vi "Signal Processing.vi"(0 "Vessel in":refnum<class "Vessel.lvclass">, 5 "error in (no error)":errorcluster) -> (14 "Vessel out":refnum<class "Vessel.lvclass">, 19 "error out":errorcluster)   [LabVIEW 2014, in "Vessel.lvclass"]
uses:
  Vessel.lvclass
  Vessel.lvclass/Vessel.ctl
  Supervisor/Supervisor.lvclass
  Sensor/Sensor.lvclass
panel:
  in  "T_dvl":dbl[](array[numeric])=[0.0, 0.0, 45.0]
  in  "Manual Sensor\nPosition Override":bool
  in  "r_dvl":dbl[](array[numeric])=[0.46, -0.5, 0.0]
  in  "r_tp":dbl[](array[numeric])=[1.35, 0.15, 0.0]
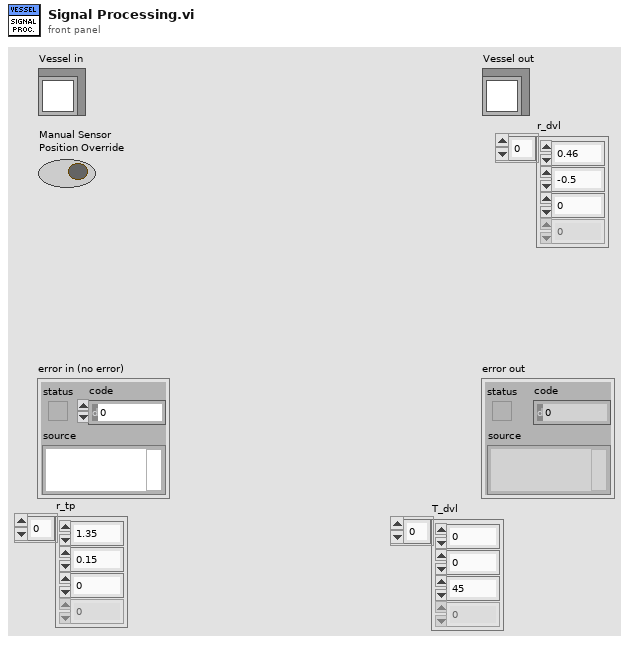
[diagram p1: front panel]
types:
  T1 = cluster{"Measured":cluster{"Eta":dbl[], "Nu":dbl[], "Eta Dot":dbl[], "Nu Dot":dbl[]}, "Estimated":cluster{"Eta":dbl[], "Nu":dbl[], "Eta Dot":dbl[], "Nu Dot":dbl[]}, "Desired":cluster{"Eta":dbl[], "Nu":dbl[], "Eta Dot":dbl[], "Nu Dot":dbl[]}, "Previous Desired":cluster{"Eta":dbl[], "Nu":dbl[], "Eta Dot":dbl[], "Nu Dot":dbl[]}, "tau":dbl[], "Altitude":cluster{"Measured":dbl, "Estimated":dbl, "Desired":dbl, "Previous Desired":dbl, "Approximated":dbl, "grad F":dbl[]}, "rpm":dbl[], "Attitude":cluster{"Theta Measured":dbl[], "Theta Estimated":dbl[], "Omega Measured":dbl[], "Omega Estimated":dbl[], "Gyro Bias":dbl[]}}
  T2 = cluster{"Set Origin":bool, "New WP":bool, "Types of Change":enum16{"Current NED", "Change NED"}, "Make Change":bool, "Optimal Heading":bool, "New SetPoint":cluster{"North":dbl, "East":dbl, "Depth":dbl, "Heading":dbl}, "Update Reference":cluster{"Mode Change":bool, "Current Position":dbl[]}, "Go":bool, "Go heading":bool}
  T3 = cluster{"Sensor Drop Out":dbl[], "Sensor Health":bool[]}
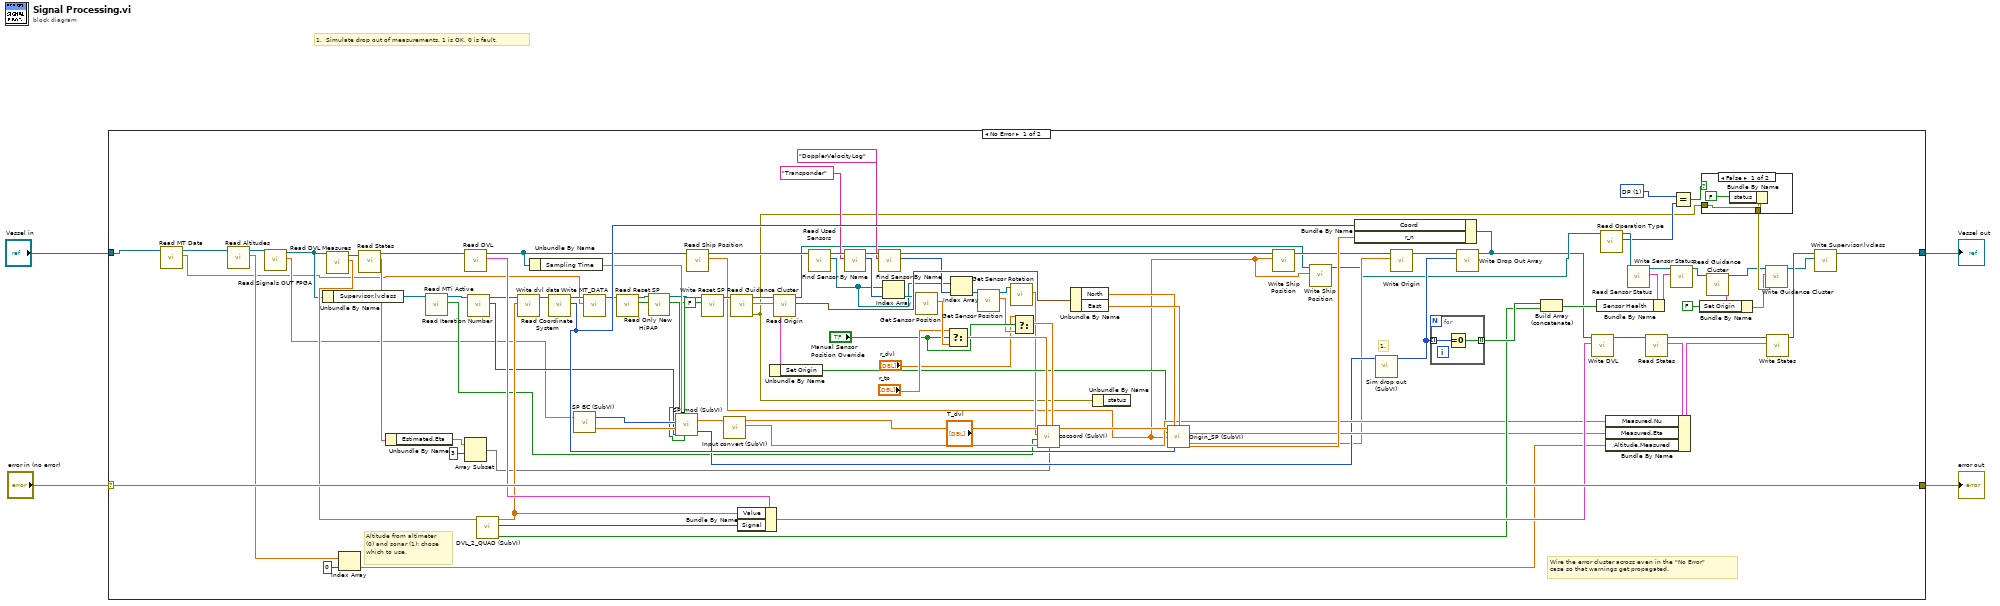
[diagram p0: block diagram]
diagram:
  # "1.  Simulate drop out of measurements. 1 is OK, 0 is fault."
  n1 = case shown="No Error" "error in (no error)" {
    selector: "error in (no error)" -> [w110 w118]
    tunnel: [w110 w118] -> w3
    tunnel: [w103 w117] -> w1
    tunnel: "Vessel in" -> [w18 w117]
    frame No Error {
      w84 = u16 1 items=["Tracking", "DP", "Joystick"] ("Operation Type")
      # "1."
      # "Altitude from altimeter (0) and sonar (1): chose which to use."
      # "Wire the error cluster across even in the \"No Error\"\ncase so that warnings get propagated."
      n2 = call-dynamic "Read MT Data.vi"("Vessel in"=w18) -> ("MT Data"=w16:sgl[], "Vessel out"=w17:refnum<class "Vessel.lvclass">)  [unwired: 8 in, 1 out]
      n3 = call-dynamic "Read Altitudes.vi"("Vessel in"=w17) -> ("Altitudes"=w19:dbl[], "Vessel out"=w20:refnum<class "Vessel.lvclass">)  [unwired: 8 in, 1 out]
      n4 = call-dynamic "Read Signals OUT FPGA.vi"("Vessel in"=w20) -> ("Signals OUT"=w21:dbl[], "Vessel out"=w22:refnum<class "Vessel.lvclass">)  [unwired: 8 in, 1 out]
      n5 = Unbundle By Name(w22) -> ("Supervisor.lvclass"=w37:refnum<class "Supervisor.lvclass">)
      n6 = call-dynamic "Read DVL Measures.vi"("Vessel in"=w22) -> ("DVL Measures"=w23:dbl[], "Vessel out"=w24:refnum<class "Vessel.lvclass">)  [unwired: 8 in, 1 out]
      n7 = Index Array(array=w19, index=0) -> (element=w47:dbl)
      n8 = call-dynamic "Read States.vi"("Vessel in"=w24) -> ("States"=w41:T1, "Vessel out"=w42:refnum<class "Vessel.lvclass">)  [unwired: 8 in, 1 out]
      n9 = Unbundle By Name(w41) -> ("Estimated.Eta"=w40:dbl[])
      n10 = call-dynamic "Read MTi Active.vi"("Supervisor in"=w37) -> ("MTi Active"=w35:bool, "Supervisor out"=w36:refnum<class "Supervisor.lvclass">)  [unwired: 8 in, 1 out]
      n11 = Array Subset(array=w40, index=3) -> (w38:dbl[])  [unwired: 1 in]
      n12 = call-dynamic "Read DVL.vi"("Vessel in"=w42) -> ("DVL"=w93:cluster{"Value":dbl[], "Signal":i32[]}, "Vessel out"=w13:refnum<class "Vessel.lvclass">)  [unwired: 8 in, 1 out]
      n13 = call-dynamic "Read Iteration Number.vi"("Supervisor in"=w36) -> ("Iteration Number"=w73:i32, "Supervisor out"=w74:refnum<class "Supervisor.lvclass">)  [unwired: 8 in, 1 out]
      n14 = call "DVL_2_QUAD (SubVI).vi"("dvl_m"=w23) -> ("DVL OK"=w81:bool[], "dvl_sig"=w102:i32[], "DVL"=w88:dbl[])  [unwired: 8 in]
      n15 = call-dynamic "Write dvl data.vi"("dvl data"=w88, "Supervisor in"=w74) -> ("Supervisor out"=w89:refnum<class "Supervisor.lvclass">)  [unwired: 8 in, 1 out]
      n16 = Unbundle By Name(w13) -> ("Sampling Time"=w77:dbl)
      n17 = call-dynamic "Read Coordinate System.vi"("Supervisor in"=w89) -> ("Coordinate System"=w94:u16, "Supervisor out"=w79:refnum<class "Supervisor.lvclass">)  [unwired: 8 in, 1 out]
      n18 = call "SP BC (SubVI).vi"("raw signals"=w21) -> ("pro signals"=w76:dbl[], "do"=w78:i16[])  [unwired: 1 in]
      n19 = call-dynamic "Write MT_DATA.vi"("MT_DATA"=w16, "Supervisor in"=w79) -> ("Supervisor out"=w71:refnum<class "Supervisor.lvclass">)  [unwired: 8 in, 1 out]
      n20 = call-dynamic "Read Reset SP.vi"("Supervisor in"=w71) -> ("Reset SP"=w69:bool, "Supervisor out"=w70:refnum<class "Supervisor.lvclass">)  [unwired: 8 in, 1 out]
      n21 = call-dynamic "Read Only New HiPAP.vi"("Supervisor in"=w70) -> ("Only New HiPAP"=w72:bool, "Supervisor out"=w67:refnum<class "Supervisor.lvclass">)  [unwired: 8 in, 1 out]
      n22 = call "SP_mod (SubVI).vi"("Only new HiPaP updates to obs"=w72, "Reset SP"=w69, "loop it"=w73, "Raw in"=w76, "Drop-Out In"=w78, "dt"=w77) -> ("Drop-Out Out"=w44:i16[], "Raw out"=w75:dbl[])
      n23 = call-dynamic "Read Ship Position.vi"("Vessel in"=w13) -> ("Ship Position"=w5:dbl[], "Vessel out"=w10:refnum<class "Vessel.lvclass">)  [unwired: 8 in, 1 out]
      n24 = call-dynamic "Write Reset SP.vi"("Reset SP"=FALSE, "Supervisor in"=w67) -> ("Supervisor out"=w68:refnum<class "Supervisor.lvclass">)  [unwired: 8 in, 1 out]
      n25 = call "Input convert (SubVI).vi"("Signals in"=w75) -> ("Nu mes"=w92:dbl[], "Eta mes"=w91:dbl[])  [unwired: 8 in, 1 out]
      n26 = call-dynamic "Read Guidance Cluster.vi"("Supervisor in"=w68) -> ("error out"=w9:errorcluster, "Guidance Cluster"=w30:T2, "Supervisor out"=w99:refnum<class "Supervisor.lvclass">)  [unwired: 8 in]
      n27 = Bundle By Name(cluster=w93, "Value"=w88, "Signal"=w102) -> (w101:cluster{"Value":dbl[], "Signal":i32[]})
      n28 = Unbundle By Name(w30) -> ("Set Origin"=w29:bool)
      n29 = call-dynamic "Read Origin.vi"("Supervisor in"=w99) -> ("Origin"=w98:cluster{"North":dbl, "East":dbl}, "Supervisor out"=w8:refnum<class "Supervisor.lvclass">)  [unwired: 8 in, 1 out]
      n30 = call "Read Used Sensors.vi"("Vessel in"=w10) -> ("Used Sensors"=w53:refnum<class "Sensor.lvclass">[], "Vessel out"=w63:refnum<class "Vessel.lvclass">)  [unwired: 8 in, 1 out]
      n31 = call "Find Sensor By Name.vi"("Sensor Name"="Transponder", "Vessel in"=w63) -> ("Sensor Index"=w61:i32, "Vessel out"=w62:refnum<class "Vessel.lvclass">)  [unwired: 7 in, 1 out]
      n32 = call "Find Sensor By Name.vi"("Sensor Name"="DopplerVelocityLog", "Vessel in"=w62) -> ("Sensor Index"=w54:i32, "Vessel out"=w11:refnum<class "Vessel.lvclass">)  [unwired: 7 in, 1 out]
      n33 = Index Array(array=w53, index=w61) -> (element=w60:refnum<class "Sensor.lvclass">)
      n34 = call-dynamic "Get Sensor Position.vi"("Sensor in"=w60) -> ("Sensor Position"=w59:dbl[])  [unwired: 8 in, 2 out]
      n35 = Select(t="r_tp", s="Manual Sensor\nPosition Override", f=w59) -> (s? t:f=w55:dbl[])
      n36 = Index Array(array=w53, index=w54) -> (element=w52:refnum<class "Sensor.lvclass">)
      n37 = call-dynamic "Get Sensor Position.vi"("Sensor in"=w52) -> ("Sensor Position"=w50:dbl[], "Sensor out"=w45:refnum<class "Sensor.lvclass">)  [unwired: 8 in, 1 out]
      n38 = call-dynamic "Get Sensor Rotation.vi"("Sensor in"=w45) -> ("Sensor Rotation"=w28:dbl[])  [unwired: 8 in, 2 out]
      n39 = Select(t="r_dvl", s="Manual Sensor\nPosition Override", f=w50) -> (s? t:f=w48:dbl[])
      n40 = call "cocoord (SubVI).vi"("r_dvl"=w48, "Attitude est"=w38, "r_tp"=w55, "nu"=w92, "MTi active"=w35, "T_dvl"=w28, "eta"=w91) -> ("nu_out"=w65:dbl[], "eta_out"=w90:dbl[])  [unwired: 3 in]
      n41 = Unbundle By Name(w98) -> ("North"=w96:dbl, "East"=w97:dbl)
      n42 = Unbundle By Name(w9) -> ()  [unwired: 1 out]
      n43 = call "Origin_SP (SubVI).vi"("eta in"=w90, "North O"=w96, "East O"=w97, "Set Orign"=w29, "eta in ship"=w5, "Ring"=w94) -> ("eta (local)"=w64:dbl[], "Origin"=w14:dbl[], "r_n"=w95:dbl[])  [unwired: 6 in, 1 out]
      n44 = call-dynamic "Write Ship Position.vi"("Ship Position"=w5, "Vessel in"=w11) -> ("Vessel out"=w12:refnum<class "Vessel.lvclass">)  [unwired: 8 in, 1 out]
      n45 = call-dynamic "Write Ship Position.vi"("Ship Position"=w5, "Supervisor in"=w8) -> ("Supervisor out"=w7:refnum<class "Supervisor.lvclass">)  [unwired: 8 in, 1 out]
      n46 = call "Sim drop out (SubVI).vi"("Drop-Out Out in"=w44) -> ("Drop-Out Out out"=w43:i16[])  [unwired: 10 in]
      n47 = call-dynamic "Write Origin.vi"("Origin"=w14, "Vessel in"=w12) -> ("Vessel out"=w15:refnum<class "Vessel.lvclass">)  [unwired: 8 in, 1 out]
      n48 = for {
        tunnel: [w115] -> w82 mode=indexing
        tunnel: w43 -> [w116] mode=indexing
        n49 = Equal To 0?(x=w116) -> (x = 0?=w115:bool)
      }
      n50 = call-dynamic "Write Drop Out Array.vi"("Drop Out Array"=w43, "Vessel in"=w15) -> ("Vessel out"=w6:refnum<class "Vessel.lvclass">)  [unwired: 8 in, 1 out]
      n51 = Bundle By Name(cluster=w6, "Coord"=w94, "r_n"=w95) -> ()  [unwired: 1 out]
      n52 = Build Array (concatenate)(w82, w81) -> (w80:bool[])
      n53 = call-dynamic "Write DVL.vi"("DVL"=w101, "Vessel in"=w6) -> ("Vessel out"=w100:refnum<class "Vessel.lvclass">)  [unwired: 8 in, 1 out]
      n54 = call-dynamic "Read Operation Type.vi"("Supervisor in"=w7) -> ("Operation Type"=w85:u16, "Supervisor out"=w86:refnum<class "Supervisor.lvclass">)  [unwired: 8 in, 1 out]
      n55 = call-dynamic "Read Sensor Status.vi"("Supervisor in"=w86) -> ("Sensor Status"=w109:T3, "Supervisor out"=w108:refnum<class "Supervisor.lvclass">)  [unwired: 8 in, 1 out]
      n56 = Bundle By Name(cluster=w109, "Sensor Health"=w80) -> (w33:T3)
      n57 = call-dynamic "Read States.vi"("Vessel in"=w100) -> ("States"=w107:T1, "Vessel out"=w105:refnum<class "Vessel.lvclass">)  [unwired: 8 in, 1 out]
      n58 = Bundle By Name(cluster=w107, "Measured.Nu"=w65, "Measured.Eta"=w64, "Altitude.Measured"=w47) -> (w106:T1)
      n59 = call-dynamic "Write Sensor Status.vi"("Sensor Status"=w33, "Supervisor in"=w108) -> ("Supervisor out"=w32:refnum<class "Supervisor.lvclass">)  [unwired: 8 in, 1 out]
      n60 = Equal?(x=w84, y=w85) -> (x = y?=w83:bool)
      n61 = case shown="False" w83 {
        tunnel: w9 -> [w112 w114]
        tunnel: [w111 w114] -> w34
        frame False {
          n62 = Bundle By Name(cluster=w112, "status"=FALSE ("Set Origin")) -> (w111:errorcluster)
        }
        frame True {
        }
      }
      n63 = call-dynamic "Read Guidance Cluster.vi"("Supervisor in"=w32) -> ("Guidance Cluster"=w27:T2, "Supervisor out"=w31:refnum<class "Supervisor.lvclass">)  [unwired: 8 in, 1 out]
      n64 = Bundle By Name(cluster=w27, "Set Origin"=FALSE) -> (w25:T2)
      n65 = call-dynamic "Write Guidance Cluster.vi"("error in (no error)"=w34, "Guidance Cluster"=w25, "Supervisor in"=w31) -> ("Supervisor out"=w87:refnum<class "Supervisor.lvclass">)  [unwired: 7 in, 1 out]
      n66 = call-dynamic "Write States.vi"("States"=w106, "Vessel in"=w105) -> ("Vessel out"=w104:refnum<class "Vessel.lvclass">)  [unwired: 8 in, 1 out]
      n67 = call "Write Supervisor.lvclass.vi"("Supervisor.lvclass"=w87, "Vessel in"=w104) -> ("Vessel out"=w103:refnum<class "Vessel.lvclass">)  [unwired: 8 in, 1 out]
    }
    frame Error {
    }
  }
  "error out" <- w3
  "Vessel out" <- w1
